vi "加标回收率计算.vi"(11 "参数":T1) -> (2 "加标后理论浓度":dbl, 3 "参数 out":T1)   [LabVIEW 2016, in "质控单元V2.lvlib"]
panel:
  out "电子表格字符串":string
  out "V1(mL)":dbl
  out "R":dbl
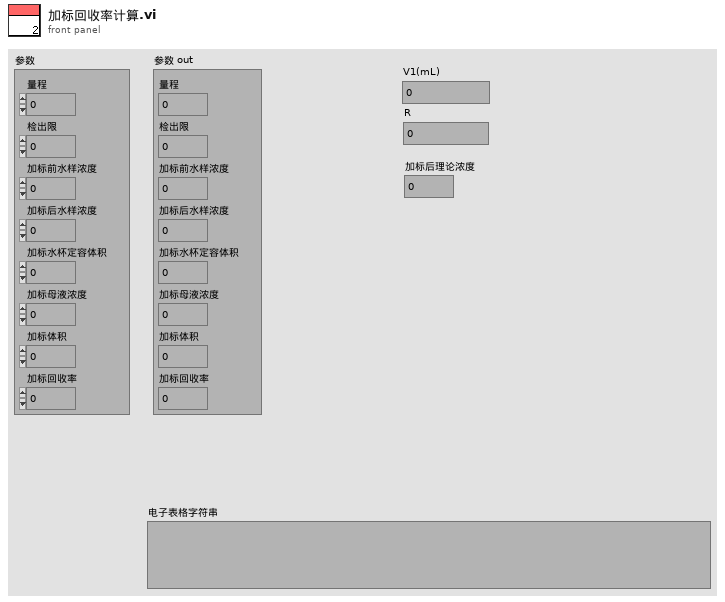
[diagram p1: front panel]
types:
  T1 = cluster{"量程":dbl, "检出限":dbl, "加标前水样浓度":dbl, "加标后水样浓度":dbl, "加标水杯定容体积":dbl, "加标母液浓度":dbl, "加标体积":dbl, "加标回收率":dbl}
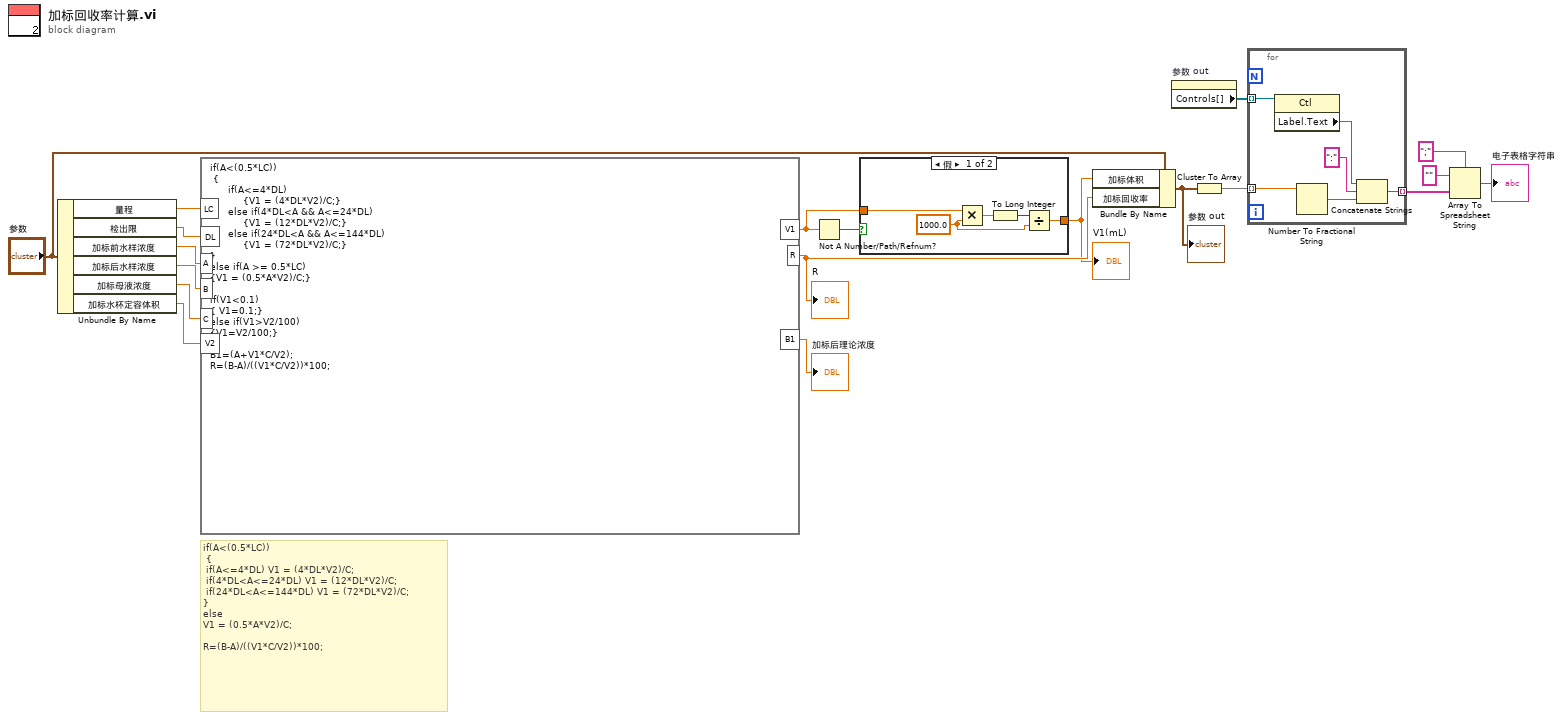
[diagram p0: block diagram]
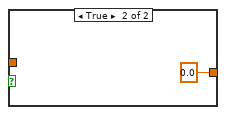
[diagram p2: hidden frame]
diagram:
  # "if(A<(0.5*LC))\n {\n if(A<=4*DL) V1 = (4*DL*V2)/C;\n if(4*DL<A<=24*DL) V1 = (12*DL*V2)/C;\n if(24*DL<A<=144*DL) V1 = (72*DL*V2)/C;\n}\nelse\nV1 = (0.5*A*V2)/C;\n\nR=(B-A)/((V1*C/V2))*100;"
  n1 = Unbundle By Name("参数") -> ("量程"=w16:dbl, "检出限"=w15:dbl, "加标前水样浓度"=w19:dbl, "加标后水样浓度"=w18:dbl, "加标母液浓度"=w17:dbl, "加标水杯定容体积"=w14:dbl)
  n2 = formula code="if(A<(0.5*LC))\n {\n      if(A<=4*DL) \n           {V1 = (4*DL*V2)/C;}\n      else if(4*DL<A && A<=24*DL) \n           {V1 = (12*DL*V2)/C;}\n      else if(24*DL<A && A<=144*DL) \n           {V1 = (72*DL*V2)/C;}\n}\nelse if(A >= 0.5*LC)\n{V1 = (0.5*A*V2)/C;}\n\nif(V1<0.1)\n{ V1=0.1;}\nelse if(V1>V2/100)\n{V1=V2/100;}\n\nB1=(A+V1*C/V2);\nR=(B-A)/((V1*C/V2))*100;"("A"=w19, "B"=w18, "C"=w17, "V2"=w14, "LC"=w16, "DL"=w15) -> ("R"=w12:dbl, "V1"=w9:dbl, "B1"=→"加标后理论浓度":dbl)
  "R" <- w12
  n3 = Not A Number/Path/Refnum?(number/path/refnum=w9) -> (NaN/Path/Refnum?=w10:bool)
  n4 = case shown="假" w10 {
    tunnel: [w20 0.0 ("V1(mL)")] -> w1
    tunnel: w9 -> [w24 _]
    frame False {
      w21 = 1000.0 ("y")
      n5 = Multiply(x=w24, y=w21) -> (x*y=w23:dbl)
      n6 = To Long Integer(number=w23) -> (32bit integer=w22:i32)
      n7 = Divide(x=w22, y=w21) -> (x/y=w20:dbl)
    }
    frame True {
    }
  }
  "V1(mL)" <- w1
  n8 = Bundle By Name(cluster="参数", "加标体积"=w1, "加标回收率"=w12) -> (w8:T1)
  "参数 out" <- w8
  n9 = property on="参数 out" class="Clust (严格)"() -> ("Controls[]"=w4:refnum<vi>[])  [unwired: 2 in, 2 out]
  n10 = Cluster To Array(cluster=w8) -> (array=w3:dbl[])
  n11 = for {
    tunnel: w4 -> [w31] mode=indexing
    tunnel: w3 -> [w29] mode=indexing
    tunnel: [w26] -> w2 mode=indexing
    n12 = property class="Ctl"(reference=w31) -> ("Label.Text"=w30:string)  [unwired: 1 in, 2 out]
    n13 = Number To Fractional String(number=w29) -> (F-format string=w27:string)  [unwired: 3 in]
    n14 = Concatenate Strings(w30, ":" ("字符串"), w27) -> (w26:string)
  }
  n15 = Array To Spreadsheet String(delimiter (Tab)=";" ("分隔符(Tab)"), array=w2, 3:"") -> (spreadsheet string=→"电子表格字符串":string)
